vi "test Configuration.vi"(8 "error in (no error)":errorcluster, 11 "BM Configuration in":refnum<class "BM Configuration.lvclass">) -> (0 "error out":errorcluster, 3 "BM Configuration out":refnum<class "BM Configuration.lvclass">)   [LabVIEW 2016, in "BM Configuration.lvclass"]
uses:
  BM Configuration.lvclass
  1553 Board/1553 Board.lvclass
  PPLs/FPGA Interface.lvlibp/FPGA Interface/FPGA Interface.lvclass
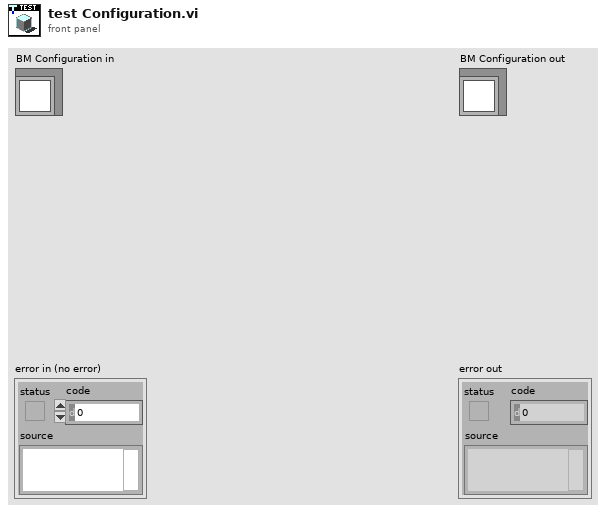
[diagram p1: front panel]
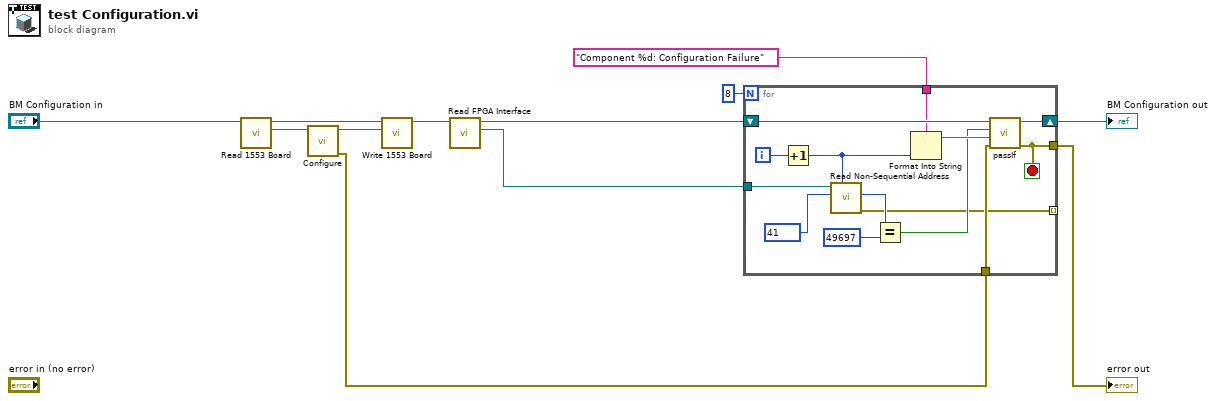
[diagram p0: block diagram]
diagram:
  n1 = call-dynamic "Read 1553 Board.vi"("1553 Test in"="BM Configuration in") -> ("1553 Board"=w7:refnum<class "1553 Board.lvclass">, "1553 Test out"=w8:refnum<class "BM Configuration.lvclass">)  [unwired: 8 in, 1 out]
  n2 = call-dynamic "Configure.vi"("1553 Board in"=w7) -> ("error out"=w1:errorcluster, "1553 Board out"=w6:refnum<class "1553 Board.lvclass">)  [unwired: 9 in]
  n3 = call-dynamic "Write 1553 Board.vi"("1553 Board"=w6, "1553 Test in"=w8) -> ("1553 Test out"=w5:refnum<class "BM Configuration.lvclass">)  [unwired: 8 in, 1 out]
  n4 = call-dynamic "Read FPGA Interface.vi"("1553 Test in"=w5) -> ("FPGA Interface"=w2:refnum<class "FPGA Interface.lvclass">, "1553 Test out"=w3:refnum<class "BM Configuration.lvclass">)  [unwired: 8 in, 1 out]
  n5 = for {
    N: 8 -> [_]
    tunnel: w2 -> [w26]
    shift-right: [w22] -> w9
    shift-left: w3 -> [w23]
    tunnel: "Component %d: Configuration Failure" ("custom report message (\"\")") -> [w21]
    tunnel: w1 -> [w16]
    tunnel: [w15] -> w10
    tunnel: [w14] -> _ mode=indexing
    i -> [w25]
    stop <- w15 stop-if-true
    n6 = Increment(x=w25) -> (x+1=w20:i32)
    n7 = call-dynamic "Read Non-Sequential Address.vi"("Target IC (1-8)"=w20, "Address"=u16 41, "FPGA Interface in"=w26) -> ("error out"=w14:errorcluster, "Data"=w18:u16)  [unwired: 7 in]
    n8 = Equal?(x=w18, y=u16 49697) -> (x = y?=w17:bool)
    n9 = Format Into String(format string=w21, w20) -> (resulting string=w19:string)  [unwired: 2 in, 1 out]
    n10 = call-dynamic "passIf.vi"("error in (no error)"=w16, "message (\"\")"=w19, "pass"=w17, "TestCase in"=w23) -> ("error out"=w15:errorcluster, "TestCase out"=w22:refnum<class "BM Configuration.lvclass">)  [unwired: 6 in]
  }
  "error out" <- w10
  "BM Configuration out" <- w9
